vi "Wifi_Data.vi"(0 "GEA2 Reference In":refnum<k24>, 11 "Error In":errorcluster) -> (3 "Wifi Network State":string, 4 "GEA2 Reference Out":refnum<k24>, 6 "Mac Address":string, 8 "Wifi Network Name":string, 10 "Wifi Password":string, 15 "Error Out":errorcluster)   [LabVIEW 2023]
uses:
  D:/Common/LabVIEW GEA2 Toolkit/source/GEA3 DLL Source/GeaCommunication.dll
  Common/LabVIEW GEA2 Toolkit/source/GEA3 DLL Source/GeaCommunication.dll
  Common/LabVIEW GEA2 Toolkit/GEA3/type defs/Source_Destination.ctl
  Common/LabVIEW GEA2 Toolkit/GEA3/type defs/ERD Read Data In.ctl
  Common/LabVIEW GEA2 Toolkit/GEA3/library/GEA2_Toolkit.lvlib
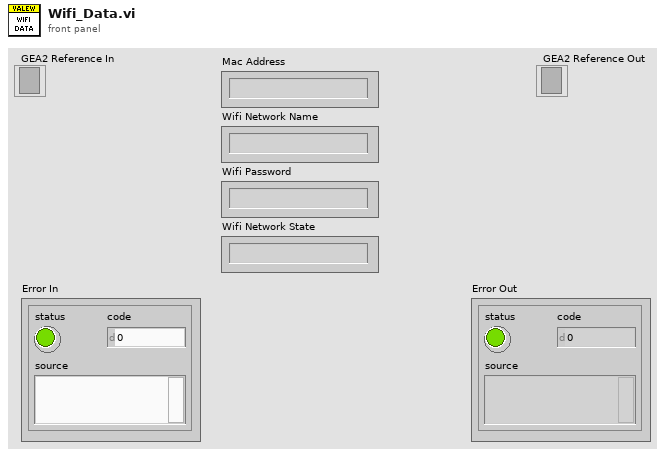
[diagram p1: front panel]
types:
  T1 = typedef "ERD Read Data In.ctl" = cluster{"ERD Number":u16, "Data Type":enum16{"string", "boolean", "uint8_t", "uint16_t", "uint32_t", "uint64_t", "int8_t", "int16_t", "int32_t", "int64_t"}}
  T2 = typedef "Source_Destination.ctl" = cluster{"Source":u8, "Destination":u8}
  T3 = cluster{"ERD Data Out[0]":cluster{"ERD Number":u16, "Data":string}, "ERD Data Out[1]":cluster{"ERD Number":u16, "Data":string}, "ERD Data Out[2]":cluster{"ERD Number":u16, "Data":string}, "ERD Data Out[3]":cluster{"ERD Number":u16, "Data":string}, "ERD Data Out[4]":cluster{"ERD Number":u16, "Data":string}, "ERD Data Out[5]":cluster{"ERD Number":u16, "Data":string}, "ERD Data Out[6]":cluster{"ERD Number":u16, "Data":string}, "ERD Data Out[7]":cluster{"ERD Number":u16, "Data":string}, "ERD Data Out[8]":cluster{"ERD Number":u16, "Data":string}}
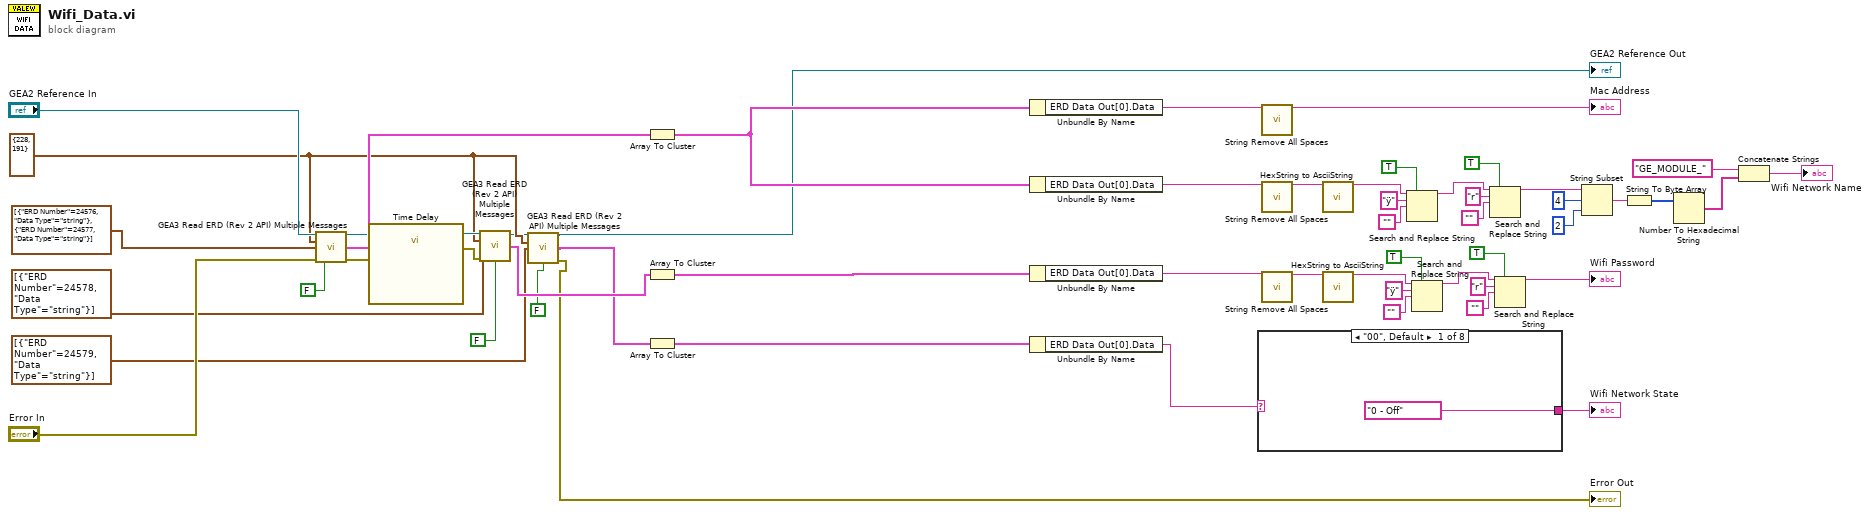
[diagram p0: block diagram]
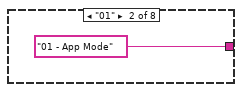
[diagram p2: hidden frame]
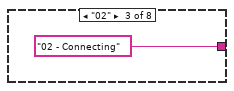
[diagram p3: hidden frame]
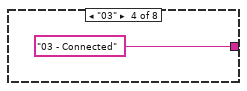
[diagram p4: hidden frame]
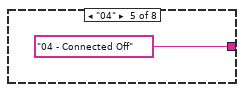
[diagram p5: hidden frame]
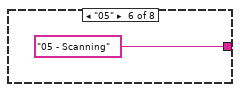
[diagram p6: hidden frame]
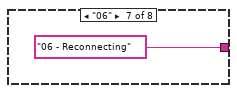
[diagram p7: hidden frame]
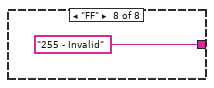
[diagram p8: hidden frame]
diagram:
  w15 = T2 {"Source"=228, "Destination"=191} ("GEA Inputs")
  n1 = call "GEA3 Read ERD (Rev 2 API) Multiple Messages.vi"("GEA2 Reference In"="GEA2 Reference In", "GEA Inputs"=w15, "Read ERD List"=T1[] [{"ERD Number"=24576, "Data Type"=enum."string"}, {"ERD Number"=24577, "Data Type"=enum."string"}], "Error In"="Error In", "Verify ERD Response?"=FALSE) -> ("GEA2 Reference Out"=w21:refnum<k24>, "ERD Data Out"=w51:cluster{"ERD Number":u16, "Data":string}[], "Error Out"=w20:errorcluster)  [unwired: 7 in, 1 out]
  n2 = call "Time Delay"("error in (no error)"=w20) -> ("error out"=w19:errorcluster)  [unwired: 10 in]
  n3 = call "GEA3 Read ERD (Rev 2 API) Multiple Messages.vi"("GEA2 Reference In"=w21, "GEA Inputs"=w15, "Read ERD List"=T1[] [{"ERD Number"=24578, "Data Type"=enum."string"}], "Error In"=w19, "Verify ERD Response?"=FALSE) -> ("GEA2 Reference Out"=w9:refnum<k24>, "ERD Data Out"=w24:cluster{"ERD Number":u16, "Data":string}[])  [unwired: 7 in, 2 out]
  n4 = call "GEA3 Read ERD (Rev 2 API) Multiple Messages.vi"("GEA2 Reference In"=w9, "GEA Inputs"=w15, "Read ERD List"=T1[] [{"ERD Number"=24579, "Data Type"=enum."string"}], "Verify ERD Response?"=FALSE) -> ("GEA2 Reference Out"=→"GEA2 Reference Out":refnum<k24>, "ERD Data Out"=w11:cluster{"ERD Number":u16, "Data":string}[], "Error Out"=→"Error Out":errorcluster)  [unwired: 8 in, 1 out]
  n5 = Array To Cluster(array=w51) -> (cluster=w50:T3)
  n6 = Array To Cluster(array=w24) -> (cluster=w23:T3)
  n7 = Array To Cluster(array=w11) -> (cluster=w17:T3)
  n8 = Unbundle By Name(w50) -> ("ERD Data Out[0].Data"=w31:string)
  n9 = Unbundle By Name(w50) -> ("ERD Data Out[0].Data"=w29:string)
  n10 = Unbundle By Name(w23) -> ("ERD Data Out[0].Data"=w27:string)
  n11 = Unbundle By Name(w17) -> ("ERD Data Out[0].Data"=w26:string)
  n12 = case shown="\"00\", Default" w26 {
    tunnel: ["0 - Off" "01 - App Mode" "02 - Connecting" "03 - Connected" "04 - Connected Off" "05 - Scanning" "06 - Reconnecting" "255 - Invalid"] -> w25
    frame "00", Default {
    }
    frame "01" {
    }
    frame "02" {
    }
    frame "03" {
    }
    frame "04" {
    }
    frame "05" {
    }
    frame "06" {
    }
    frame "FF" {
    }
  }
  "Wifi Network State" <- w25
  n13 = call "String Remove All Spaces.vi"("Input String"=w31) -> ("Spaces Removed"=→"Mac Address":string)  [unwired: 13 in, 1 out]
  n14 = call "String Remove All Spaces.vi"("Input String"=w29) -> ("Spaces Removed"=w49:string)  [unwired: 13 in, 1 out]
  n15 = call "String Remove All Spaces.vi"("Input String"=w27) -> ("Spaces Removed"=w40:string)  [unwired: 13 in, 1 out]
  n16 = call "HexString to AsciiString.vi"("Hex String"=w49) -> ("ASCII String"=w45:string)  [unwired: 13 in, 1 out]
  n17 = call "HexString to AsciiString.vi"("Hex String"=w40) -> ("ASCII String"=w36:string)  [unwired: 13 in, 1 out]
  n18 = Search and Replace String(replace all?=TRUE ("replace all? (F)"), input string=w45, search string="ÿ", replace string="") -> (result string=w42:string)  [unwired: 4 in, 3 out]
  n19 = Search and Replace String(replace all?=TRUE ("replace all? (F)"), input string=w36, search string="ÿ", replace string="") -> (result string=w33:string)  [unwired: 4 in, 3 out]
  n20 = Search and Replace String(replace all?=TRUE ("replace all? (F)"), input string=w42, search string="r", replace string="") -> (result string=w8:string)  [unwired: 4 in, 3 out]
  n21 = Search and Replace String(replace all?=TRUE ("replace all? (F)"), input string=w33, search string="r", replace string="") -> (result string=→"Wifi Password":string)  [unwired: 4 in, 3 out]
  n22 = String Subset(string=w8, offset (0)=4, length (rest)=2 ("length (rest)")) -> (substring=w5:string)
  n23 = String To Byte Array(string=w5) -> (unsigned byte array=w4:u8[])
  n24 = Number To Hexadecimal String(2:w4) -> (0:w3:string[])  [unwired: 1 in]
  n25 = Concatenate Strings("GE_MODULE_" ("string"), w3) -> (→"Wifi Network Name":string)
